vi "ReadIni.vi"(1 "configuration file path":path=path "E:/LabVIEW/福尔达/AppData") -> ()   [LabVIEW 2018]
uses:
  <vilib>/Utility/config.llb/Read Key (String).vi
  <vilib>/Utility/config.llb/Read Key (Double).vi
  <vilib>/Utility/config.llb/Read Key (U32).vi
  <vilib>/Utility/config.llb/NI_LVConfig.lvlib
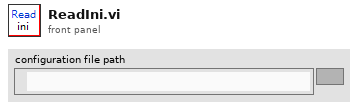
[diagram p1: front panel]
types:
  T1 = typedef "NI_LVConfig.lvlib/Config Data RefNum.ctl" = refnum<k1>
  T2 = cluster{"轮盘预压力":sgl, "泄漏量上限":sgl, "压力上限":sgl, "压力下限":sgl, "风门闭电压上限":sgl, "风门闭电压下限":sgl, "风门开电压上限":sgl, "风门开电压下限":sgl, "LED电流上限":sgl, "LED电流下限":sgl, "气压稳定时间":sgl, "伺服速度":sgl}
  T3 = cluster{"选择":enum16{"Fx", "Fy", "Fz", "Mx", "My", "Mz"}, "系数":sgl, "上限":sgl, "下限":sgl, "Ymax":dbl, "Ymin":dbl, "点数":dbl, "锁系数x":sgl, "锁上限":sgl, "锁下限":sgl, "锁系数+":sgl, "起点":dbl, "终点":dbl, "锁起点":dbl, "锁终点":dbl}
  T4 = cluster{"选择":enum16{"Fx", "Fy", "Fz", "Mx", "My", "Mz"}, "系数":sgl, "上限":sgl, "下限":sgl, "Ymax":dbl, "Ymin":dbl, "点数":dbl, "起点":dbl, "终点":dbl}
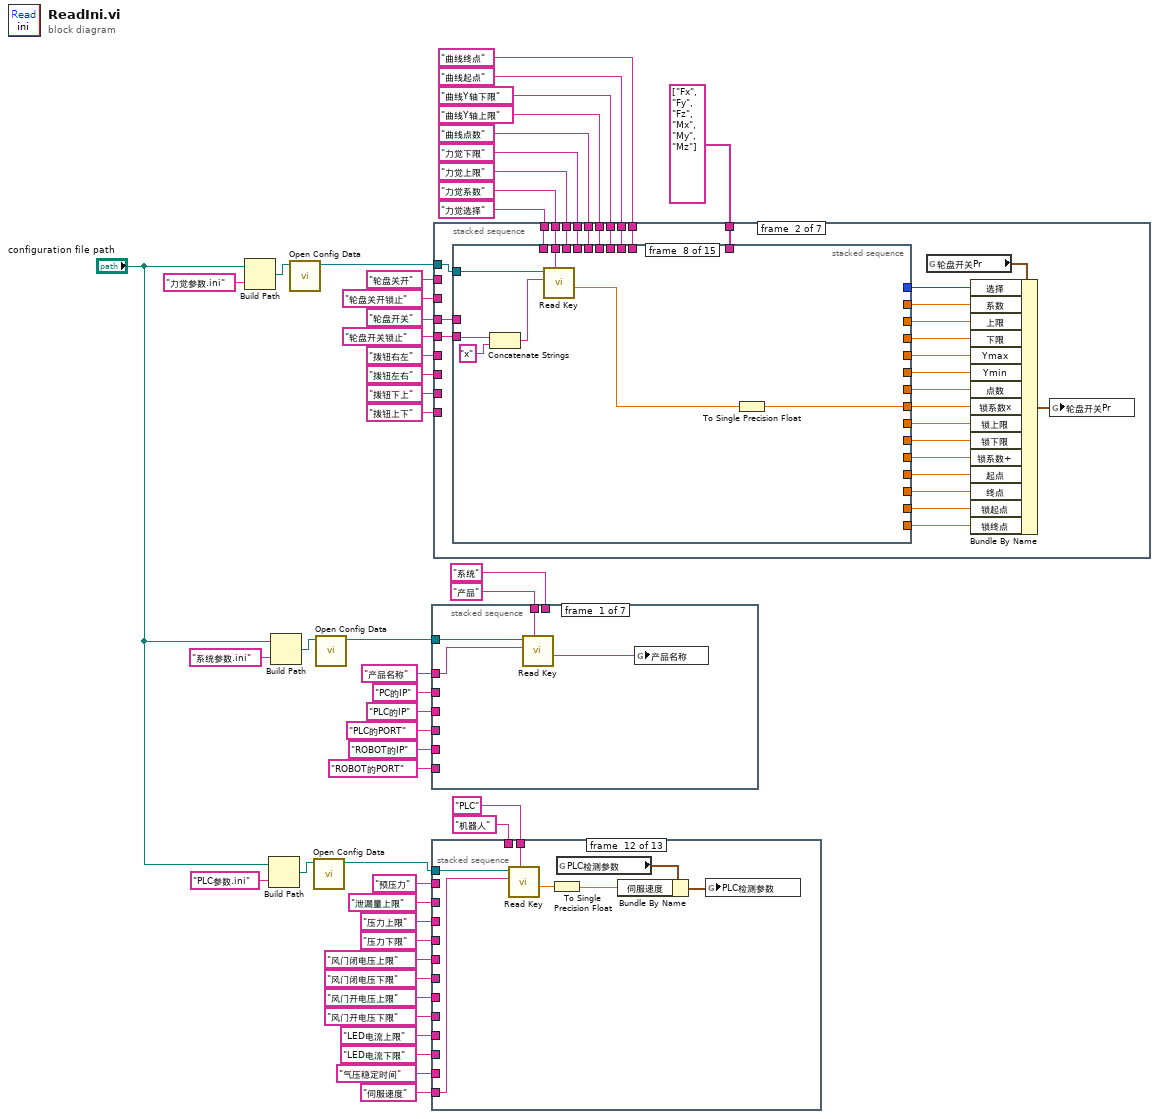
[diagram p0: block diagram]
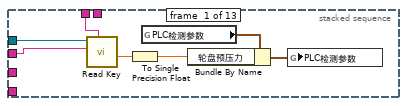
[diagram p2: hidden frame]
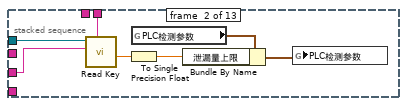
[diagram p3: hidden frame]
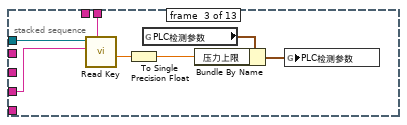
[diagram p4: hidden frame]
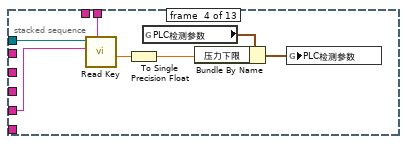
[diagram p5: hidden frame]
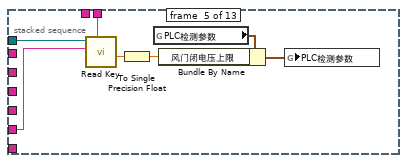
[diagram p6: hidden frame]
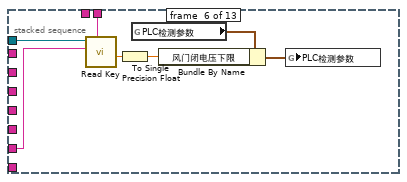
[diagram p7: hidden frame]
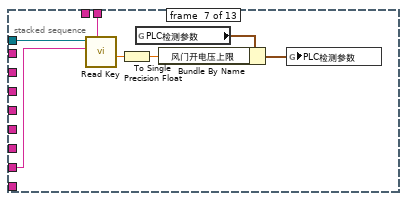
[diagram p8: hidden frame]
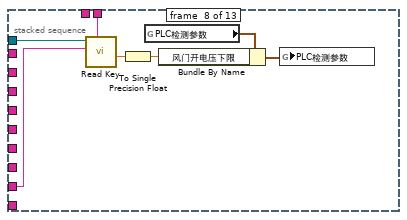
[diagram p9: hidden frame]
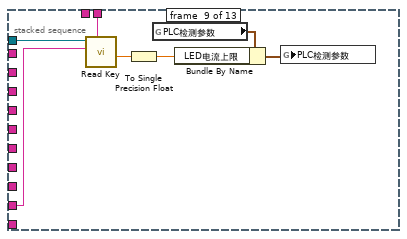
[diagram p10: hidden frame]
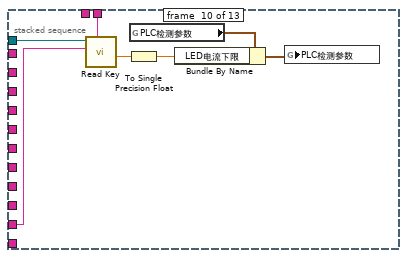
[diagram p11: hidden frame]
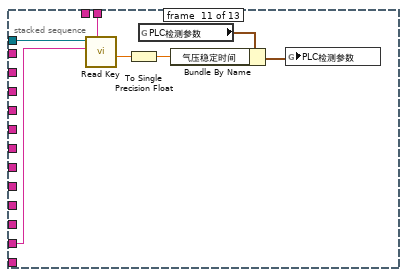
[diagram p12: hidden frame]
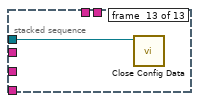
[diagram p13: hidden frame]
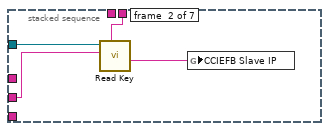
[diagram p14: hidden frame]
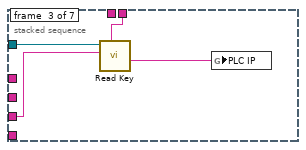
[diagram p15: hidden frame]
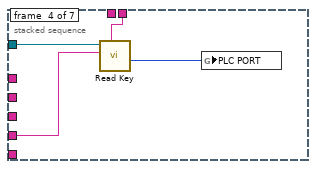
[diagram p16: hidden frame]
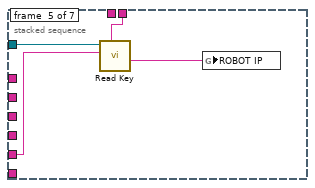
[diagram p17: hidden frame]
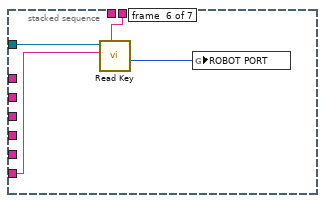
[diagram p18: hidden frame]
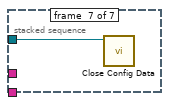
[diagram p19: hidden frame]
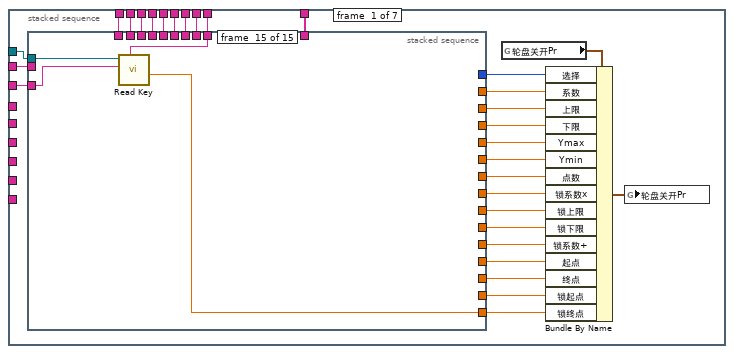
[diagram p20: hidden frame]
diagram:
  n1 = Build Path(base path="configuration file path", name or relative path="力觉参数.ini" ("名称或相对路径")) -> (appended path=w31:path)
  n2 = Build Path(base path="configuration file path", name or relative path="PLC参数.ini" ("名称或相对路径")) -> (appended path=w16:path)
  n3 = Build Path(base path="configuration file path", name or relative path="系统参数.ini" ("名称或相对路径")) -> (appended path=w29:path)
  n4 = call <vilib>:"Open Config Data.vi"("configuration file path"=w31) -> ("refnum"=w47:T1)  [unwired: 8 in, 2 out]
  n5 = call <vilib>:"Open Config Data.vi"("configuration file path"=w16) -> ("refnum"=w13:T1)  [unwired: 8 in, 2 out]
  n6 = call <vilib>:"Open Config Data.vi"("configuration file path"=w29) -> ("refnum"=w27:T1)  [unwired: 8 in, 2 out]
  n7 = stacked-sequence {
    tunnel: w27 -> [w53 w57 w61 w65 w69 w73 w75]
    tunnel: "产品" -> [w52 _ _ _ _ _ _]
    tunnel: "PC的IP" -> [_ w56 _ _ _ _ _]
    tunnel: "产品名称" -> [w51 _ _ _ _ _ _]
    tunnel: "PLC的IP" -> [_ _ w60 _ _ _ _]
    tunnel: "PLC的PORT" -> [_ _ _ w64 _ _ _]
    tunnel: "ROBOT的IP" -> [_ _ _ _ w68 _ _]
    tunnel: "ROBOT的PORT" -> [_ _ _ _ _ w72 _]
    tunnel: "系统" -> [_ w55 w59 w63 w67 w71 _]
    frame #0 {
      n8 = call-poly <vilib>:"Read Key.vi"("section"=w52, "key"=w51, "refnum"=w53) -> ("value"=w54:string)  [unwired: 5 in, 3 out]
      n9 = global write "全局 1.vi" "产品名称"(w54) -> ()
    }
    frame #1 {
      n10 = call-poly <vilib>:"Read Key.vi"("section"=w55, "key"=w56, "refnum"=w57) -> ("value"=w58:string)  [unwired: 5 in, 3 out]
      n11 = global write "全局 1.vi" "CCIEFB Slave IP"(w58) -> ()
    }
    frame #2 {
      n12 = call-poly <vilib>:"Read Key.vi"("section"=w59, "key"=w60, "refnum"=w61) -> ("value"=w62:string)  [unwired: 5 in, 3 out]
      n13 = global write "全局 1.vi" "PLC IP"(w62) -> ()
    }
    frame #3 {
      n14 = call-poly <vilib>:"Read Key.vi"("section"=w63, "key"=w64, "refnum"=w65) -> ("value"=w66:u32)  [unwired: 5 in, 3 out]
      n15 = global write "全局 1.vi" "PLC PORT"(w66) -> ()
    }
    frame #4 {
      n16 = call-poly <vilib>:"Read Key.vi"("section"=w67, "key"=w68, "refnum"=w69) -> ("value"=w70:string)  [unwired: 5 in, 3 out]
      n17 = global write "全局 1.vi" "ROBOT IP"(w70) -> ()
    }
    frame #5 {
      n18 = call-poly <vilib>:"Read Key.vi"("section"=w71, "key"=w72, "refnum"=w73) -> ("value"=w74:u32)  [unwired: 5 in, 3 out]
      n19 = global write "全局 1.vi" "ROBOT PORT"(w74) -> ()
    }
    frame #6 {
      n20 = call <vilib>:"Close Config Data.vi"("refnum"=w75) -> ()  [unwired: 9 in, 2 out]
    }
  }
  n21 = stacked-sequence {
    tunnel: "机器人" -> [w78 _ _ _ _ _ _ _ _ _ _ _ _]
    tunnel: "PLC" -> [_ w85 w92 w99 w106 w113 w120 w127 w134 w141 w148 w155 _]
    tunnel: w13 -> [w77 w84 w91 w98 w105 w112 w119 w126 w133 w140 w147 w154 w160]
    tunnel: "预压力" -> [w76 _ _ _ _ _ _ _ _ _ _ _ _]
    tunnel: "泄漏量上限" -> [_ w83 _ _ _ _ _ _ _ _ _ _ _]
    tunnel: "压力上限" -> [_ _ w90 _ _ _ _ _ _ _ _ _ _]
    tunnel: "压力下限" -> [_ _ _ w97 _ _ _ _ _ _ _ _ _]
    tunnel: "风门闭电压上限" -> [_ _ _ _ w104 _ _ _ _ _ _ _ _]
    tunnel: "风门闭电压下限" -> [_ _ _ _ _ w111 _ _ _ _ _ _ _]
    tunnel: "风门开电压上限" -> [_ _ _ _ _ _ w118 _ _ _ _ _ _]
    tunnel: "风门开电压下限" -> [_ _ _ _ _ _ _ w125 _ _ _ _ _]
    tunnel: "LED电流上限" -> [_ _ _ _ _ _ _ _ w132 _ _ _ _]
    tunnel: "LED电流下限" -> [_ _ _ _ _ _ _ _ _ w139 _ _ _]
    tunnel: "气压稳定时间" -> [_ _ _ _ _ _ _ _ _ _ w146 _ _]
    tunnel: "伺服速度" -> [_ _ _ _ _ _ _ _ _ _ _ w153 _]
    frame #0 {
      n22 = call-poly <vilib>:"Read Key.vi"("section"=w78, "key"=w76, "refnum"=w77) -> ("value"=w82:dbl)  [unwired: 5 in, 3 out]
      n23 = To Single Precision Float(number=w82) -> (single precision float=w81:sgl)
      n24 = global read "全局 1.vi" "PLC检测参数"() -> (w79:T2)
      n25 = Bundle By Name(cluster=w79, "轮盘预压力"=w81) -> (w80:T2)
      n26 = global write "全局 1.vi" "PLC检测参数"(w80) -> ()
    }
    frame #1 {
      n27 = call-poly <vilib>:"Read Key.vi"("section"=w85, "key"=w83, "refnum"=w84) -> ("value"=w89:dbl)  [unwired: 5 in, 3 out]
      n28 = To Single Precision Float(number=w89) -> (single precision float=w88:sgl)
      n29 = global read "全局 1.vi" "PLC检测参数"() -> (w86:T2)
      n30 = Bundle By Name(cluster=w86, "泄漏量上限"=w88) -> (w87:T2)
      n31 = global write "全局 1.vi" "PLC检测参数"(w87) -> ()
    }
    frame #2 {
      n32 = call-poly <vilib>:"Read Key.vi"("section"=w92, "key"=w90, "refnum"=w91) -> ("value"=w96:dbl)  [unwired: 5 in, 3 out]
      n33 = To Single Precision Float(number=w96) -> (single precision float=w95:sgl)
      n34 = global read "全局 1.vi" "PLC检测参数"() -> (w93:T2)
      n35 = Bundle By Name(cluster=w93, "压力上限"=w95) -> (w94:T2)
      n36 = global write "全局 1.vi" "PLC检测参数"(w94) -> ()
    }
    frame #3 {
      n37 = call-poly <vilib>:"Read Key.vi"("section"=w99, "key"=w97, "refnum"=w98) -> ("value"=w103:dbl)  [unwired: 5 in, 3 out]
      n38 = To Single Precision Float(number=w103) -> (single precision float=w102:sgl)
      n39 = global read "全局 1.vi" "PLC检测参数"() -> (w100:T2)
      n40 = Bundle By Name(cluster=w100, "压力下限"=w102) -> (w101:T2)
      n41 = global write "全局 1.vi" "PLC检测参数"(w101) -> ()
    }
    frame #4 {
      n42 = call-poly <vilib>:"Read Key.vi"("section"=w106, "key"=w104, "refnum"=w105) -> ("value"=w110:dbl)  [unwired: 5 in, 3 out]
      n43 = To Single Precision Float(number=w110) -> (single precision float=w109:sgl)
      n44 = global read "全局 1.vi" "PLC检测参数"() -> (w107:T2)
      n45 = Bundle By Name(cluster=w107, "风门闭电压上限"=w109) -> (w108:T2)
      n46 = global write "全局 1.vi" "PLC检测参数"(w108) -> ()
    }
    frame #5 {
      n47 = call-poly <vilib>:"Read Key.vi"("section"=w113, "key"=w111, "refnum"=w112) -> ("value"=w117:dbl)  [unwired: 5 in, 3 out]
      n48 = To Single Precision Float(number=w117) -> (single precision float=w116:sgl)
      n49 = global read "全局 1.vi" "PLC检测参数"() -> (w114:T2)
      n50 = Bundle By Name(cluster=w114, "风门闭电压下限"=w116) -> (w115:T2)
      n51 = global write "全局 1.vi" "PLC检测参数"(w115) -> ()
    }
    frame #6 {
      n52 = call-poly <vilib>:"Read Key.vi"("section"=w120, "key"=w118, "refnum"=w119) -> ("value"=w124:dbl)  [unwired: 5 in, 3 out]
      n53 = To Single Precision Float(number=w124) -> (single precision float=w123:sgl)
      n54 = global read "全局 1.vi" "PLC检测参数"() -> (w121:T2)
      n55 = Bundle By Name(cluster=w121, "风门开电压上限"=w123) -> (w122:T2)
      n56 = global write "全局 1.vi" "PLC检测参数"(w122) -> ()
    }
    frame #7 {
      n57 = call-poly <vilib>:"Read Key.vi"("section"=w127, "key"=w125, "refnum"=w126) -> ("value"=w131:dbl)  [unwired: 5 in, 3 out]
      n58 = To Single Precision Float(number=w131) -> (single precision float=w130:sgl)
      n59 = global read "全局 1.vi" "PLC检测参数"() -> (w128:T2)
      n60 = Bundle By Name(cluster=w128, "风门开电压下限"=w130) -> (w129:T2)
      n61 = global write "全局 1.vi" "PLC检测参数"(w129) -> ()
    }
    frame #8 {
      n62 = call-poly <vilib>:"Read Key.vi"("section"=w134, "key"=w132, "refnum"=w133) -> ("value"=w138:dbl)  [unwired: 5 in, 3 out]
      n63 = To Single Precision Float(number=w138) -> (single precision float=w137:sgl)
      n64 = global read "全局 1.vi" "PLC检测参数"() -> (w135:T2)
      n65 = Bundle By Name(cluster=w135, "LED电流上限"=w137) -> (w136:T2)
      n66 = global write "全局 1.vi" "PLC检测参数"(w136) -> ()
    }
    frame #9 {
      n67 = call-poly <vilib>:"Read Key.vi"("section"=w141, "key"=w139, "refnum"=w140) -> ("value"=w145:dbl)  [unwired: 5 in, 3 out]
      n68 = To Single Precision Float(number=w145) -> (single precision float=w144:sgl)
      n69 = global read "全局 1.vi" "PLC检测参数"() -> (w142:T2)
      n70 = Bundle By Name(cluster=w142, "LED电流下限"=w144) -> (w143:T2)
      n71 = global write "全局 1.vi" "PLC检测参数"(w143) -> ()
    }
    frame #10 {
      n72 = call-poly <vilib>:"Read Key.vi"("section"=w148, "key"=w146, "refnum"=w147) -> ("value"=w152:dbl)  [unwired: 5 in, 3 out]
      n73 = To Single Precision Float(number=w152) -> (single precision float=w151:sgl)
      n74 = global read "全局 1.vi" "PLC检测参数"() -> (w149:T2)
      n75 = Bundle By Name(cluster=w149, "气压稳定时间"=w151) -> (w150:T2)
      n76 = global write "全局 1.vi" "PLC检测参数"(w150) -> ()
    }
    frame #11 {
      n77 = call-poly <vilib>:"Read Key.vi"("section"=w155, "key"=w153, "refnum"=w154) -> ("value"=w159:dbl)  [unwired: 5 in, 3 out]
      n78 = To Single Precision Float(number=w159) -> (single precision float=w158:sgl)
      n79 = global read "全局 1.vi" "PLC检测参数"() -> (w156:T2)
      n80 = Bundle By Name(cluster=w156, "伺服速度"=w158) -> (w157:T2)
      n81 = global write "全局 1.vi" "PLC检测参数"(w157) -> ()
    }
    frame #12 {
      n82 = call <vilib>:"Close Config Data.vi"("refnum"=w160) -> ()  [unwired: 9 in, 2 out]
    }
  }
  n83 = stacked-sequence {
    tunnel: string[] ["Fx", "Fy", "Fz", "Mx", "My", "Mz"] -> [w190 w294 w391 w456 w521 w586 _]
    tunnel: "轮盘关开" -> [w185 _ _ _ _ _ _]
    tunnel: "轮盘开关" -> [_ w266 _ _ _ _ _]
    tunnel: w47 -> [w189 w293 w390 w455 w520 w585 w629]
    tunnel: "力觉选择" -> [w184 w289 w386 w451 w516 w581 _]
    tunnel: "力觉系数" -> [w183 w288 w385 w450 w515 w580 _]
    tunnel: "力觉上限" -> [w182 w287 w384 w449 w514 w579 _]
    tunnel: "力觉下限" -> [w181 w286 w383 w448 w513 w578 _]
    tunnel: "曲线点数" -> [w180 w285 w382 w447 w512 w577 _]
    tunnel: "曲线Y轴上限" -> [w179 w284 w381 w446 w511 w576 _]
    tunnel: "曲线Y轴下限" -> [w178 w283 w380 w445 w510 w575 _]
    tunnel: "轮盘关开锁止" -> [w168 _ _ _ _ _ _]
    tunnel: "轮盘开关锁止" -> [_ w265 _ _ _ _ _]
    tunnel: "拨钮右左" -> [_ _ w377 _ _ _ _]
    tunnel: "拨钮左右" -> [_ _ _ w434 _ _ _]
    tunnel: "拨钮下上" -> [_ _ _ _ w499 _ _]
    tunnel: "拨钮上下" -> [_ _ _ _ _ w564 _]
    tunnel: "曲线起点" -> [w177 w282 w379 w444 w509 w574 _]
    tunnel: "曲线终点" -> [w176 w281 w378 w443 w508 w573 _]
    frame #0 {
      n84 = stacked-sequence {
        tunnel: w190 -> [w197 _ _ _ _ _ _ _ _ _ _ _ _ _ _]
        tunnel: w185 -> [w195 w202 w207 w212 w216 w220 w224 _ _ _ _ w249 w253 _ _]
        tunnel: w189 -> [w194 w201 w206 w211 w215 w219 w223 w231 w236 w241 w248 w252 w256 w260 w264]
        tunnel: [w193 _ _ _ _ _ _ _ _ _ _ _ _ _ _] -> w187
        tunnel: w184 -> [w191 _ _ _ _ _ _ _ _ _ _ _ _ _ _]
        tunnel: w183 -> [_ w200 _ _ _ _ _ w230 _ _ w242 _ _ _ _]
        tunnel: w182 -> [_ _ w203 _ _ _ _ _ w233 _ _ _ _ _ _]
        tunnel: w181 -> [_ _ _ w208 _ _ _ _ _ w237 _ _ _ _ _]
        tunnel: w180 -> [_ _ _ _ _ _ w222 _ _ _ _ _ _ _ _]
        tunnel: w179 -> [_ _ _ _ w214 _ _ _ _ _ _ _ _ _ _]
        tunnel: w178 -> [_ _ _ _ _ w217 _ _ _ _ _ _ _ _ _]
        tunnel: w177 -> [_ _ _ _ _ _ _ _ _ _ _ w251 _ w257 _]
        tunnel: w176 -> [_ _ _ _ _ _ _ _ _ _ _ _ w254 _ w263]
        tunnel: [_ w198 _ _ _ _ _ _ _ _ _ _ _ _ _] -> w175
        tunnel: [_ _ w204 _ _ _ _ _ _ _ _ _ _ _ _] -> w174
        tunnel: [_ _ _ w209 _ _ _ _ _ _ _ _ _ _ _] -> w173
        tunnel: [_ _ _ _ w213 _ _ _ _ _ _ _ _ _ _] -> w172
        tunnel: [_ _ _ _ _ w218 _ _ _ _ _ _ _ _ _] -> w171
        tunnel: [_ _ _ _ _ _ w221 _ _ _ _ _ _ _ _] -> w170
        tunnel: [_ _ _ _ _ _ _ w226 _ _ _ _ _ _ _] -> w169
        tunnel: w168 -> [_ _ _ _ _ _ _ w229 w232 w239 w245 _ _ w258 w262]
        tunnel: [_ _ _ _ _ _ _ _ w234 _ _ _ _ _ _] -> w167
        tunnel: [_ _ _ _ _ _ _ _ _ w238 _ _ _ _ _] -> w166
        tunnel: [_ _ _ _ _ _ _ _ _ _ w246 _ _ _ _] -> w165
        tunnel: [_ _ _ _ _ _ _ _ _ _ _ w250 _ _ _] -> w164
        tunnel: [_ _ _ _ _ _ _ _ _ _ _ _ w255 _ _] -> w163
        tunnel: [_ _ _ _ _ _ _ _ _ _ _ _ _ w259 _] -> w162
        tunnel: [_ _ _ _ _ _ _ _ _ _ _ _ _ _ w261] -> w161
        frame #0 {
          n85 = call-poly <vilib>:"Read Key.vi"("section"=w191, "key"=w195, "refnum"=w194) -> ("value"=w196:string)  [unwired: 5 in, 3 out]
          n86 = Search 1D Array(1D array=w197, element=w196) -> (index of element=w192:i32)  [unwired: 1 in]
          n87 = To Unsigned Word Integer(number=w192) -> (unsigned 16bit integer=w193:u16)
        }
        frame #1 {
          n88 = call-poly <vilib>:"Read Key.vi"("section"=w200, "key"=w202, "refnum"=w201) -> ("value"=w199:dbl)  [unwired: 5 in, 3 out]
          n89 = To Single Precision Float(number=w199) -> (single precision float=w198:sgl)
        }
        frame #2 {
          n90 = call-poly <vilib>:"Read Key.vi"("section"=w203, "key"=w207, "refnum"=w206) -> ("value"=w205:dbl)  [unwired: 5 in, 3 out]
          n91 = To Single Precision Float(number=w205) -> (single precision float=w204:sgl)
        }
        frame #3 {
          n92 = call-poly <vilib>:"Read Key.vi"("section"=w208, "key"=w212, "refnum"=w211) -> ("value"=w210:dbl)  [unwired: 5 in, 3 out]
          n93 = To Single Precision Float(number=w210) -> (single precision float=w209:sgl)
        }
        frame #4 {
          n94 = call-poly <vilib>:"Read Key.vi"("section"=w214, "key"=w216, "refnum"=w215) -> ("value"=w213:dbl)  [unwired: 5 in, 3 out]
        }
        frame #5 {
          n95 = call-poly <vilib>:"Read Key.vi"("section"=w217, "key"=w220, "refnum"=w219) -> ("value"=w218:dbl)  [unwired: 5 in, 3 out]
        }
        frame #6 {
          n96 = call-poly <vilib>:"Read Key.vi"("section"=w222, "key"=w224, "refnum"=w223) -> ("value"=w221:dbl)  [unwired: 5 in, 3 out]
        }
        frame #7 {
          n97 = Concatenate Strings(w229, "x") -> (w228:string)
          n98 = call-poly <vilib>:"Read Key.vi"("section"=w230, "key"=w228, "refnum"=w231) -> ("value"=w225:dbl)  [unwired: 5 in, 3 out]
          n99 = To Single Precision Float(number=w225) -> (single precision float=w226:sgl)
        }
        frame #8 {
          n100 = call-poly <vilib>:"Read Key.vi"("section"=w233, "key"=w232, "refnum"=w236) -> ("value"=w235:dbl)  [unwired: 5 in, 3 out]
          n101 = To Single Precision Float(number=w235) -> (single precision float=w234:sgl)
        }
        frame #9 {
          n102 = call-poly <vilib>:"Read Key.vi"("section"=w237, "key"=w239, "refnum"=w241) -> ("value"=w240:dbl)  [unwired: 5 in, 3 out]
          n103 = To Single Precision Float(number=w240) -> (single precision float=w238:sgl)
        }
        frame #10 {
          n104 = Concatenate Strings(w245, "+") -> (w244:string)
          n105 = call-poly <vilib>:"Read Key.vi"("section"=w242, "key"=w244, "refnum"=w248) -> ("value"=w247:dbl)  [unwired: 5 in, 3 out]
          n106 = To Single Precision Float(number=w247) -> (single precision float=w246:sgl)
        }
        frame #11 {
          n107 = call-poly <vilib>:"Read Key.vi"("section"=w251, "key"=w249, "refnum"=w252) -> ("value"=w250:dbl)  [unwired: 5 in, 3 out]
        }
        frame #12 {
          n108 = call-poly <vilib>:"Read Key.vi"("section"=w254, "key"=w253, "refnum"=w256) -> ("value"=w255:dbl)  [unwired: 5 in, 3 out]
        }
        frame #13 {
          n109 = call-poly <vilib>:"Read Key.vi"("section"=w257, "key"=w258, "refnum"=w260) -> ("value"=w259:dbl)  [unwired: 5 in, 3 out]
        }
        frame #14 {
          n110 = call-poly <vilib>:"Read Key.vi"("section"=w263, "key"=w262, "refnum"=w264) -> ("value"=w261:dbl)  [unwired: 5 in, 3 out]
        }
      }
      n111 = global read "全局 1.vi" "轮盘关开Pr"() -> (w188:T3)
      n112 = Bundle By Name(cluster=w188, "选择"=w187, "系数"=w175, "上限"=w174, "下限"=w173, "Ymax"=w172, "Ymin"=w171, "点数"=w170, "锁系数x"=w169, "锁上限"=w167, "锁下限"=w166, "锁系数+"=w165, "起点"=w164, "终点"=w163, "锁起点"=w162, "锁终点"=w161) -> (w186:T3)
      n113 = global write "全局 1.vi" "轮盘关开Pr"(w186) -> ()
    }
    frame #1 {
      n114 = stacked-sequence {
        tunnel: w294 -> [w301 _ _ _ _ _ _ _ _ _ _ _ _ _ _]
        tunnel: w293 -> [w299 w306 w311 w316 w320 w324 w328 w335 w340 w345 w352 w356 w360 w364 w368]
        tunnel: [w298 _ _ _ _ _ _ _ _ _ _ _ _ _ _] -> w291
        tunnel: w289 -> [w296 _ _ _ _ _ _ _ _ _ _ _ _ _ _]
        tunnel: w288 -> [_ w305 _ _ _ _ _ w334 _ _ w347 _ _ _ _]
        tunnel: w287 -> [_ _ w308 _ _ _ _ _ w337 _ _ _ _ _ _]
        tunnel: w286 -> [_ _ _ w313 _ _ _ _ _ w342 _ _ _ _ _]
        tunnel: w285 -> [_ _ _ _ _ _ w327 _ _ _ _ _ _ _ _]
        tunnel: w284 -> [_ _ _ _ w319 _ _ _ _ _ _ _ _ _ _]
        tunnel: w283 -> [_ _ _ _ _ w322 _ _ _ _ _ _ _ _ _]
        tunnel: w282 -> [_ _ _ _ _ _ _ _ _ _ _ w355 _ w362 _]
        tunnel: w281 -> [_ _ _ _ _ _ _ _ _ _ _ _ w358 _ w367]
        tunnel: [_ w303 _ _ _ _ _ _ _ _ _ _ _ _ _] -> w280
        tunnel: [_ _ w309 _ _ _ _ _ _ _ _ _ _ _ _] -> w279
        tunnel: [_ _ _ w314 _ _ _ _ _ _ _ _ _ _ _] -> w278
        tunnel: [_ _ _ _ w318 _ _ _ _ _ _ _ _ _ _] -> w277
        tunnel: [_ _ _ _ _ w323 _ _ _ _ _ _ _ _ _] -> w276
        tunnel: [_ _ _ _ _ _ w326 _ _ _ _ _ _ _ _] -> w275
        tunnel: [_ _ _ _ _ _ _ w331 _ _ _ _ _ _ _] -> w274
        tunnel: [_ _ _ _ _ _ _ _ w338 _ _ _ _ _ _] -> w273
        tunnel: [_ _ _ _ _ _ _ _ _ w343 _ _ _ _ _] -> w272
        tunnel: [_ _ _ _ _ _ _ _ _ _ w350 _ _ _ _] -> w271
        tunnel: [_ _ _ _ _ _ _ _ _ _ _ w354 _ _ _] -> w270
        tunnel: [_ _ _ _ _ _ _ _ _ _ _ _ w359 _ _] -> w269
        tunnel: [_ _ _ _ _ _ _ _ _ _ _ _ _ w363 _] -> w268
        tunnel: [_ _ _ _ _ _ _ _ _ _ _ _ _ _ w366] -> w267
        tunnel: w266 -> [w295 w302 w307 w312 w317 w321 w325 _ _ _ _ w353 w357 _ _]
        tunnel: w265 -> [_ _ _ _ _ _ _ w329 w336 w341 w346 _ _ w361 w365]
        frame #0 {
          n115 = call-poly <vilib>:"Read Key.vi"("section"=w296, "key"=w295, "refnum"=w299) -> ("value"=w300:string)  [unwired: 5 in, 3 out]
          n116 = Search 1D Array(1D array=w301, element=w300) -> (index of element=w297:i32)  [unwired: 1 in]
          n117 = To Unsigned Word Integer(number=w297) -> (unsigned 16bit integer=w298:u16)
        }
        frame #1 {
          n118 = call-poly <vilib>:"Read Key.vi"("section"=w305, "key"=w302, "refnum"=w306) -> ("value"=w304:dbl)  [unwired: 5 in, 3 out]
          n119 = To Single Precision Float(number=w304) -> (single precision float=w303:sgl)
        }
        frame #2 {
          n120 = call-poly <vilib>:"Read Key.vi"("section"=w308, "key"=w307, "refnum"=w311) -> ("value"=w310:dbl)  [unwired: 5 in, 3 out]
          n121 = To Single Precision Float(number=w310) -> (single precision float=w309:sgl)
        }
        frame #3 {
          n122 = call-poly <vilib>:"Read Key.vi"("section"=w313, "key"=w312, "refnum"=w316) -> ("value"=w315:dbl)  [unwired: 5 in, 3 out]
          n123 = To Single Precision Float(number=w315) -> (single precision float=w314:sgl)
        }
        frame #4 {
          n124 = call-poly <vilib>:"Read Key.vi"("section"=w319, "key"=w317, "refnum"=w320) -> ("value"=w318:dbl)  [unwired: 5 in, 3 out]
        }
        frame #5 {
          n125 = call-poly <vilib>:"Read Key.vi"("section"=w322, "key"=w321, "refnum"=w324) -> ("value"=w323:dbl)  [unwired: 5 in, 3 out]
        }
        frame #6 {
          n126 = call-poly <vilib>:"Read Key.vi"("section"=w327, "key"=w325, "refnum"=w328) -> ("value"=w326:dbl)  [unwired: 5 in, 3 out]
        }
        frame #7 {
          n127 = Concatenate Strings(w329, "x") -> (w333:string)
          n128 = call-poly <vilib>:"Read Key.vi"("section"=w334, "key"=w333, "refnum"=w335) -> ("value"=w330:dbl)  [unwired: 5 in, 3 out]
          n129 = To Single Precision Float(number=w330) -> (single precision float=w331:sgl)
        }
        frame #8 {
          n130 = call-poly <vilib>:"Read Key.vi"("section"=w337, "key"=w336, "refnum"=w340) -> ("value"=w339:dbl)  [unwired: 5 in, 3 out]
          n131 = To Single Precision Float(number=w339) -> (single precision float=w338:sgl)
        }
        frame #9 {
          n132 = call-poly <vilib>:"Read Key.vi"("section"=w342, "key"=w341, "refnum"=w345) -> ("value"=w344:dbl)  [unwired: 5 in, 3 out]
          n133 = To Single Precision Float(number=w344) -> (single precision float=w343:sgl)
        }
        frame #10 {
          n134 = Concatenate Strings(w346, "+") -> (w349:string)
          n135 = call-poly <vilib>:"Read Key.vi"("section"=w347, "key"=w349, "refnum"=w352) -> ("value"=w351:dbl)  [unwired: 5 in, 3 out]
          n136 = To Single Precision Float(number=w351) -> (single precision float=w350:sgl)
        }
        frame #11 {
          n137 = call-poly <vilib>:"Read Key.vi"("section"=w355, "key"=w353, "refnum"=w356) -> ("value"=w354:dbl)  [unwired: 5 in, 3 out]
        }
        frame #12 {
          n138 = call-poly <vilib>:"Read Key.vi"("section"=w358, "key"=w357, "refnum"=w360) -> ("value"=w359:dbl)  [unwired: 5 in, 3 out]
        }
        frame #13 {
          n139 = call-poly <vilib>:"Read Key.vi"("section"=w362, "key"=w361, "refnum"=w364) -> ("value"=w363:dbl)  [unwired: 5 in, 3 out]
        }
        frame #14 {
          n140 = call-poly <vilib>:"Read Key.vi"("section"=w367, "key"=w365, "refnum"=w368) -> ("value"=w366:dbl)  [unwired: 5 in, 3 out]
        }
      }
      n141 = global read "全局 1.vi" "轮盘开关Pr"() -> (w292:T3)
      n142 = Bundle By Name(cluster=w292, "选择"=w291, "系数"=w280, "上限"=w279, "下限"=w278, "Ymax"=w277, "Ymin"=w276, "点数"=w275, "锁系数x"=w274, "锁上限"=w273, "锁下限"=w272, "锁系数+"=w271, "起点"=w270, "终点"=w269, "锁起点"=w268, "锁终点"=w267) -> (w290:T3)
      n143 = global write "全局 1.vi" "轮盘开关Pr"(w290) -> ()
    }
    frame #2 {
      n144 = stacked-sequence {
        tunnel: w391 -> [w398 _ _ _ _ _ _ _ _]
        tunnel: w390 -> [w396 w403 w408 w413 w417 w421 w425 w429 w433]
        tunnel: [w395 _ _ _ _ _ _ _ _] -> w388
        tunnel: w386 -> [w393 _ _ _ _ _ _ _ _]
        tunnel: w385 -> [_ w402 _ _ _ _ _ _ _]
        tunnel: w384 -> [_ _ w406 _ _ _ _ _ _]
        tunnel: w383 -> [_ _ _ w411 _ _ _ _ _]
        tunnel: w382 -> [_ _ _ _ _ _ w424 _ _]
        tunnel: w381 -> [_ _ _ _ w416 _ _ _ _]
        tunnel: w380 -> [_ _ _ _ _ w420 _ _ _]
        tunnel: w379 -> [_ _ _ _ _ _ _ w428 _]
        tunnel: w378 -> [_ _ _ _ _ _ _ _ w432]
        tunnel: w377 -> [w392 w399 w404 w409 w414 w418 w422 w426 w430]
        tunnel: [_ w400 _ _ _ _ _ _ _] -> w376
        tunnel: [_ _ w405 _ _ _ _ _ _] -> w375
        tunnel: [_ _ _ w410 _ _ _ _ _] -> w374
        tunnel: [_ _ _ _ w415 _ _ _ _] -> w373
        tunnel: [_ _ _ _ _ w419 _ _ _] -> w372
        tunnel: [_ _ _ _ _ _ w423 _ _] -> w371
        tunnel: [_ _ _ _ _ _ _ w427 _] -> w370
        tunnel: [_ _ _ _ _ _ _ _ w431] -> w369
        frame #0 {
          n145 = call-poly <vilib>:"Read Key.vi"("section"=w393, "key"=w392, "refnum"=w396) -> ("value"=w397:string)  [unwired: 5 in, 3 out]
          n146 = Search 1D Array(1D array=w398, element=w397) -> (index of element=w394:i32)  [unwired: 1 in]
          n147 = To Unsigned Word Integer(number=w394) -> (unsigned 16bit integer=w395:u16)
        }
        frame #1 {
          n148 = call-poly <vilib>:"Read Key.vi"("section"=w402, "key"=w399, "refnum"=w403) -> ("value"=w401:dbl)  [unwired: 5 in, 3 out]
          n149 = To Single Precision Float(number=w401) -> (single precision float=w400:sgl)
        }
        frame #2 {
          n150 = call-poly <vilib>:"Read Key.vi"("section"=w406, "key"=w404, "refnum"=w408) -> ("value"=w407:dbl)  [unwired: 5 in, 3 out]
          n151 = To Single Precision Float(number=w407) -> (single precision float=w405:sgl)
        }
        frame #3 {
          n152 = call-poly <vilib>:"Read Key.vi"("section"=w411, "key"=w409, "refnum"=w413) -> ("value"=w412:dbl)  [unwired: 5 in, 3 out]
          n153 = To Single Precision Float(number=w412) -> (single precision float=w410:sgl)
        }
        frame #4 {
          n154 = call-poly <vilib>:"Read Key.vi"("section"=w416, "key"=w414, "refnum"=w417) -> ("value"=w415:dbl)  [unwired: 5 in, 3 out]
        }
        frame #5 {
          n155 = call-poly <vilib>:"Read Key.vi"("section"=w420, "key"=w418, "refnum"=w421) -> ("value"=w419:dbl)  [unwired: 5 in, 3 out]
        }
        frame #6 {
          n156 = call-poly <vilib>:"Read Key.vi"("section"=w424, "key"=w422, "refnum"=w425) -> ("value"=w423:dbl)  [unwired: 5 in, 3 out]
        }
        frame #7 {
          n157 = call-poly <vilib>:"Read Key.vi"("section"=w428, "key"=w426, "refnum"=w429) -> ("value"=w427:dbl)  [unwired: 5 in, 3 out]
        }
        frame #8 {
          n158 = call-poly <vilib>:"Read Key.vi"("section"=w432, "key"=w430, "refnum"=w433) -> ("value"=w431:dbl)  [unwired: 5 in, 3 out]
        }
      }
      n159 = global read "全局 1.vi" "拨钮右左Pr"() -> (w389:T4)
      n160 = Bundle By Name(cluster=w389, "选择"=w388, "系数"=w376, "上限"=w375, "下限"=w374, "Ymax"=w373, "Ymin"=w372, "点数"=w371, "起点"=w370, "终点"=w369) -> (w387:T4)
      n161 = global write "全局 1.vi" "拨钮右左Pr"(w387) -> ()
    }
    frame #3 {
      n162 = stacked-sequence {
        tunnel: w456 -> [w463 _ _ _ _ _ _ _ _]
        tunnel: w455 -> [w461 w468 w473 w478 w482 w486 w490 w494 w498]
        tunnel: [w460 _ _ _ _ _ _ _ _] -> w453
        tunnel: w451 -> [w458 _ _ _ _ _ _ _ _]
        tunnel: w450 -> [_ w467 _ _ _ _ _ _ _]
        tunnel: w449 -> [_ _ w471 _ _ _ _ _ _]
        tunnel: w448 -> [_ _ _ w476 _ _ _ _ _]
        tunnel: w447 -> [_ _ _ _ _ _ w489 _ _]
        tunnel: w446 -> [_ _ _ _ w481 _ _ _ _]
        tunnel: w445 -> [_ _ _ _ _ w485 _ _ _]
        tunnel: w444 -> [_ _ _ _ _ _ _ w493 _]
        tunnel: w443 -> [_ _ _ _ _ _ _ _ w497]
        tunnel: [_ w465 _ _ _ _ _ _ _] -> w442
        tunnel: [_ _ w470 _ _ _ _ _ _] -> w441
        tunnel: [_ _ _ w475 _ _ _ _ _] -> w440
        tunnel: [_ _ _ _ w480 _ _ _ _] -> w439
        tunnel: [_ _ _ _ _ w484 _ _ _] -> w438
        tunnel: [_ _ _ _ _ _ w488 _ _] -> w437
        tunnel: [_ _ _ _ _ _ _ w492 _] -> w436
        tunnel: [_ _ _ _ _ _ _ _ w496] -> w435
        tunnel: w434 -> [w457 w464 w469 w474 w479 w483 w487 w491 w495]
        frame #0 {
          n163 = call-poly <vilib>:"Read Key.vi"("section"=w458, "key"=w457, "refnum"=w461) -> ("value"=w462:string)  [unwired: 5 in, 3 out]
          n164 = Search 1D Array(1D array=w463, element=w462) -> (index of element=w459:i32)  [unwired: 1 in]
          n165 = To Unsigned Word Integer(number=w459) -> (unsigned 16bit integer=w460:u16)
        }
        frame #1 {
          n166 = call-poly <vilib>:"Read Key.vi"("section"=w467, "key"=w464, "refnum"=w468) -> ("value"=w466:dbl)  [unwired: 5 in, 3 out]
          n167 = To Single Precision Float(number=w466) -> (single precision float=w465:sgl)
        }
        frame #2 {
          n168 = call-poly <vilib>:"Read Key.vi"("section"=w471, "key"=w469, "refnum"=w473) -> ("value"=w472:dbl)  [unwired: 5 in, 3 out]
          n169 = To Single Precision Float(number=w472) -> (single precision float=w470:sgl)
        }
        frame #3 {
          n170 = call-poly <vilib>:"Read Key.vi"("section"=w476, "key"=w474, "refnum"=w478) -> ("value"=w477:dbl)  [unwired: 5 in, 3 out]
          n171 = To Single Precision Float(number=w477) -> (single precision float=w475:sgl)
        }
        frame #4 {
          n172 = call-poly <vilib>:"Read Key.vi"("section"=w481, "key"=w479, "refnum"=w482) -> ("value"=w480:dbl)  [unwired: 5 in, 3 out]
        }
        frame #5 {
          n173 = call-poly <vilib>:"Read Key.vi"("section"=w485, "key"=w483, "refnum"=w486) -> ("value"=w484:dbl)  [unwired: 5 in, 3 out]
        }
        frame #6 {
          n174 = call-poly <vilib>:"Read Key.vi"("section"=w489, "key"=w487, "refnum"=w490) -> ("value"=w488:dbl)  [unwired: 5 in, 3 out]
        }
        frame #7 {
          n175 = call-poly <vilib>:"Read Key.vi"("section"=w493, "key"=w491, "refnum"=w494) -> ("value"=w492:dbl)  [unwired: 5 in, 3 out]
        }
        frame #8 {
          n176 = call-poly <vilib>:"Read Key.vi"("section"=w497, "key"=w495, "refnum"=w498) -> ("value"=w496:dbl)  [unwired: 5 in, 3 out]
        }
      }
      n177 = global read "全局 1.vi" "拨钮左右Pr"() -> (w454:T4)
      n178 = Bundle By Name(cluster=w454, "选择"=w453, "系数"=w442, "上限"=w441, "下限"=w440, "Ymax"=w439, "Ymin"=w438, "点数"=w437, "起点"=w436, "终点"=w435) -> (w452:T4)
      n179 = global write "全局 1.vi" "拨钮左右Pr"(w452) -> ()
    }
    frame #4 {
      n180 = stacked-sequence {
        tunnel: w521 -> [w528 _ _ _ _ _ _ _ _]
        tunnel: w520 -> [w526 w533 w538 w543 w547 w551 w555 w559 w563]
        tunnel: [w525 _ _ _ _ _ _ _ _] -> w518
        tunnel: w516 -> [w523 _ _ _ _ _ _ _ _]
        tunnel: w515 -> [_ w532 _ _ _ _ _ _ _]
        tunnel: w514 -> [_ _ w536 _ _ _ _ _ _]
        tunnel: w513 -> [_ _ _ w541 _ _ _ _ _]
        tunnel: w512 -> [_ _ _ _ _ _ w554 _ _]
        tunnel: w511 -> [_ _ _ _ w546 _ _ _ _]
        tunnel: w510 -> [_ _ _ _ _ w550 _ _ _]
        tunnel: w509 -> [_ _ _ _ _ _ _ w558 _]
        tunnel: w508 -> [_ _ _ _ _ _ _ _ w562]
        tunnel: [_ w530 _ _ _ _ _ _ _] -> w507
        tunnel: [_ _ w535 _ _ _ _ _ _] -> w506
        tunnel: [_ _ _ w540 _ _ _ _ _] -> w505
        tunnel: [_ _ _ _ w545 _ _ _ _] -> w504
        tunnel: [_ _ _ _ _ w549 _ _ _] -> w503
        tunnel: [_ _ _ _ _ _ w553 _ _] -> w502
        tunnel: [_ _ _ _ _ _ _ w557 _] -> w501
        tunnel: [_ _ _ _ _ _ _ _ w561] -> w500
        tunnel: w499 -> [w522 w529 w534 w539 w544 w548 w552 w556 w560]
        frame #0 {
          n181 = call-poly <vilib>:"Read Key.vi"("section"=w523, "key"=w522, "refnum"=w526) -> ("value"=w527:string)  [unwired: 5 in, 3 out]
          n182 = Search 1D Array(1D array=w528, element=w527) -> (index of element=w524:i32)  [unwired: 1 in]
          n183 = To Unsigned Word Integer(number=w524) -> (unsigned 16bit integer=w525:u16)
        }
        frame #1 {
          n184 = call-poly <vilib>:"Read Key.vi"("section"=w532, "key"=w529, "refnum"=w533) -> ("value"=w531:dbl)  [unwired: 5 in, 3 out]
          n185 = To Single Precision Float(number=w531) -> (single precision float=w530:sgl)
        }
        frame #2 {
          n186 = call-poly <vilib>:"Read Key.vi"("section"=w536, "key"=w534, "refnum"=w538) -> ("value"=w537:dbl)  [unwired: 5 in, 3 out]
          n187 = To Single Precision Float(number=w537) -> (single precision float=w535:sgl)
        }
        frame #3 {
          n188 = call-poly <vilib>:"Read Key.vi"("section"=w541, "key"=w539, "refnum"=w543) -> ("value"=w542:dbl)  [unwired: 5 in, 3 out]
          n189 = To Single Precision Float(number=w542) -> (single precision float=w540:sgl)
        }
        frame #4 {
          n190 = call-poly <vilib>:"Read Key.vi"("section"=w546, "key"=w544, "refnum"=w547) -> ("value"=w545:dbl)  [unwired: 5 in, 3 out]
        }
        frame #5 {
          n191 = call-poly <vilib>:"Read Key.vi"("section"=w550, "key"=w548, "refnum"=w551) -> ("value"=w549:dbl)  [unwired: 5 in, 3 out]
        }
        frame #6 {
          n192 = call-poly <vilib>:"Read Key.vi"("section"=w554, "key"=w552, "refnum"=w555) -> ("value"=w553:dbl)  [unwired: 5 in, 3 out]
        }
        frame #7 {
          n193 = call-poly <vilib>:"Read Key.vi"("section"=w558, "key"=w556, "refnum"=w559) -> ("value"=w557:dbl)  [unwired: 5 in, 3 out]
        }
        frame #8 {
          n194 = call-poly <vilib>:"Read Key.vi"("section"=w562, "key"=w560, "refnum"=w563) -> ("value"=w561:dbl)  [unwired: 5 in, 3 out]
        }
      }
      n195 = global read "全局 1.vi" "拨钮下上Pr"() -> (w519:T4)
      n196 = Bundle By Name(cluster=w519, "选择"=w518, "系数"=w507, "上限"=w506, "下限"=w505, "Ymax"=w504, "Ymin"=w503, "点数"=w502, "起点"=w501, "终点"=w500) -> (w517:T4)
      n197 = global write "全局 1.vi" "拨钮下上Pr"(w517) -> ()
    }
    frame #5 {
      n198 = stacked-sequence {
        tunnel: w586 -> [w593 _ _ _ _ _ _ _ _]
        tunnel: w585 -> [w591 w598 w603 w608 w612 w616 w620 w624 w628]
        tunnel: [w590 _ _ _ _ _ _ _ _] -> w583
        tunnel: w581 -> [w588 _ _ _ _ _ _ _ _]
        tunnel: w580 -> [_ w597 _ _ _ _ _ _ _]
        tunnel: w579 -> [_ _ w601 _ _ _ _ _ _]
        tunnel: w578 -> [_ _ _ w606 _ _ _ _ _]
        tunnel: w577 -> [_ _ _ _ _ _ w619 _ _]
        tunnel: w576 -> [_ _ _ _ w611 _ _ _ _]
        tunnel: w575 -> [_ _ _ _ _ w615 _ _ _]
        tunnel: w574 -> [_ _ _ _ _ _ _ w623 _]
        tunnel: w573 -> [_ _ _ _ _ _ _ _ w627]
        tunnel: [_ w595 _ _ _ _ _ _ _] -> w572
        tunnel: [_ _ w600 _ _ _ _ _ _] -> w571
        tunnel: [_ _ _ w605 _ _ _ _ _] -> w570
        tunnel: [_ _ _ _ w610 _ _ _ _] -> w569
        tunnel: [_ _ _ _ _ w614 _ _ _] -> w568
        tunnel: [_ _ _ _ _ _ w618 _ _] -> w567
        tunnel: [_ _ _ _ _ _ _ w622 _] -> w566
        tunnel: [_ _ _ _ _ _ _ _ w626] -> w565
        tunnel: w564 -> [w587 w594 w599 w604 w609 w613 w617 w621 w625]
        frame #0 {
          n199 = call-poly <vilib>:"Read Key.vi"("section"=w588, "key"=w587, "refnum"=w591) -> ("value"=w592:string)  [unwired: 5 in, 3 out]
          n200 = Search 1D Array(1D array=w593, element=w592) -> (index of element=w589:i32)  [unwired: 1 in]
          n201 = To Unsigned Word Integer(number=w589) -> (unsigned 16bit integer=w590:u16)
        }
        frame #1 {
          n202 = call-poly <vilib>:"Read Key.vi"("section"=w597, "key"=w594, "refnum"=w598) -> ("value"=w596:dbl)  [unwired: 5 in, 3 out]
          n203 = To Single Precision Float(number=w596) -> (single precision float=w595:sgl)
        }
        frame #2 {
          n204 = call-poly <vilib>:"Read Key.vi"("section"=w601, "key"=w599, "refnum"=w603) -> ("value"=w602:dbl)  [unwired: 5 in, 3 out]
          n205 = To Single Precision Float(number=w602) -> (single precision float=w600:sgl)
        }
        frame #3 {
          n206 = call-poly <vilib>:"Read Key.vi"("section"=w606, "key"=w604, "refnum"=w608) -> ("value"=w607:dbl)  [unwired: 5 in, 3 out]
          n207 = To Single Precision Float(number=w607) -> (single precision float=w605:sgl)
        }
        frame #4 {
          n208 = call-poly <vilib>:"Read Key.vi"("section"=w611, "key"=w609, "refnum"=w612) -> ("value"=w610:dbl)  [unwired: 5 in, 3 out]
        }
        frame #5 {
          n209 = call-poly <vilib>:"Read Key.vi"("section"=w615, "key"=w613, "refnum"=w616) -> ("value"=w614:dbl)  [unwired: 5 in, 3 out]
        }
        frame #6 {
          n210 = call-poly <vilib>:"Read Key.vi"("section"=w619, "key"=w617, "refnum"=w620) -> ("value"=w618:dbl)  [unwired: 5 in, 3 out]
        }
        frame #7 {
          n211 = call-poly <vilib>:"Read Key.vi"("section"=w623, "key"=w621, "refnum"=w624) -> ("value"=w622:dbl)  [unwired: 5 in, 3 out]
        }
        frame #8 {
          n212 = call-poly <vilib>:"Read Key.vi"("section"=w627, "key"=w625, "refnum"=w628) -> ("value"=w626:dbl)  [unwired: 5 in, 3 out]
        }
      }
      n213 = global read "全局 1.vi" "拨钮上下Pr"() -> (w584:T4)
      n214 = Bundle By Name(cluster=w584, "选择"=w583, "系数"=w572, "上限"=w571, "下限"=w570, "Ymax"=w569, "Ymin"=w568, "点数"=w567, "起点"=w566, "终点"=w565) -> (w582:T4)
      n215 = global write "全局 1.vi" "拨钮上下Pr"(w582) -> ()
    }
    frame #6 {
      n216 = call <vilib>:"Close Config Data.vi"("refnum"=w629) -> ()  [unwired: 9 in, 2 out]
    }
  }
